vi "close_com.vi"(8 "error in (no error)":errorcluster) -> (0 "error out":errorcluster)   [LabVIEW 2023, in "BT-Android_interface.lvlib"]
uses:
  BT-Android_interface.lvlib
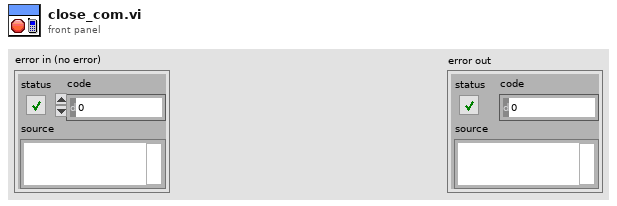
[diagram p1: front panel]
types:
  T1 = enum16{"init", "broadcast_data", "receive_data", "close", "clear_visa"}
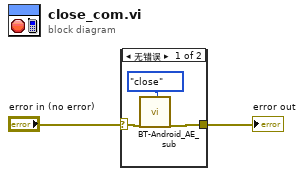
[diagram p0: block diagram]
diagram:
  n1 = case shown="无错误" "error in (no error)" {
    selector: "error in (no error)" -> [w5 w6]
    tunnel: [w4 w6] -> w1
    frame No Error {
      n2 = call "BT-Android_AE_sub.vi"("error in (no error)"=w5, "mode"=T1."close") -> ("error IO"=w4:errorcluster)  [unwired: 15 in, 2 out]
    }
    frame Error {
    }
  }
  "error out" <- w1
